vi "XIPIN_RLDRAM3_(MIG)_1_1.vi"   [LabVIEW 2017]
doc: "Memory Interface Generator for generating RLDRAM3 interfaces for Ultrascale Architecture\n------------------------------------\n<b>Need License</b> : No"
uses:
  <vilib>/rvi/XilinxIP/XIPIN_XNode/niFpgaXIPIN.xnode
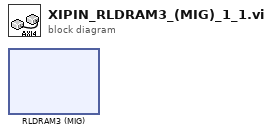
[diagram p0: block diagram]
diagram:
  n1 = xnode ("RLDRAM3 (MIG)")() -> ()
